vi "_Read - no objects.vi"() -> ()   [LabVIEW 2017]
uses:
  Global/GPIB Numbers.vi
  <vilib>/regexp/Match Regular Expression.xnode
panel:
  out "error out":errorcluster
  in  "Input Setting":dbl
  in  "Sensitivity":i8
  out "X, Y, and R array":dbl[](array[numeric])
  in  "error in (no error)":errorcluster
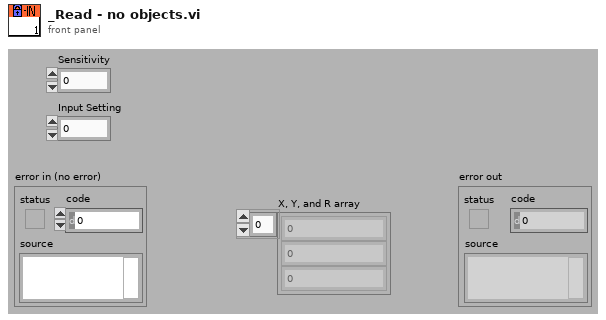
[diagram p1: front panel]
types:
  T1 = typedef "GPIB Type Def.ctl" = cluster{"Name":string, "bus":dbl, "GPIB":dbl, "GPIB as string":string, "byte":i32, "VISA Resource Name":refnum<visa-resource-name>}
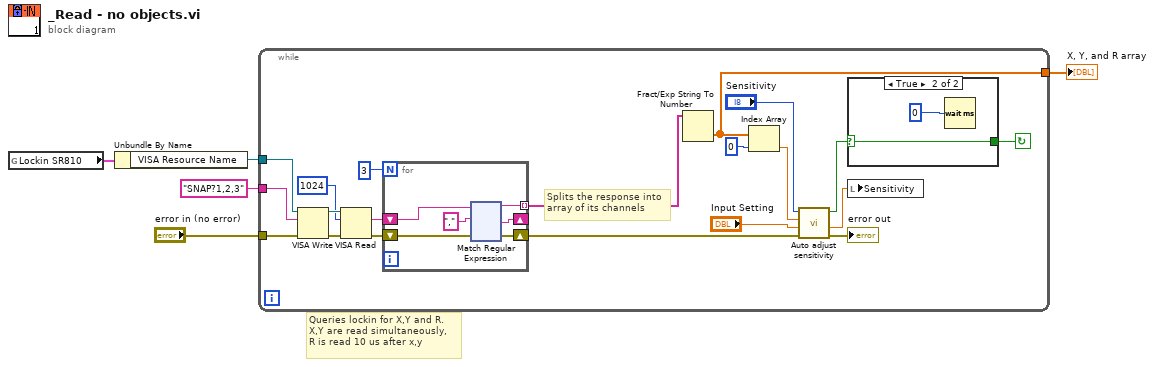
[diagram p0: block diagram]
diagram:
  # "Queries lockin for X,Y and R.\nX,Y are read simultaneously, \nR is read 10 us after x,y"
  n1 = global read "GPIB Numbers.vi" "Lockin SR810"() -> (w4:T1)
  n2 = Unbundle By Name(w4) -> ("VISA Resource Name"=w3:refnum<visa-resource-name>)
  n3 = while {
    tunnel: "SNAP?1,2,3" ("write buffer") -> [w25]
    tunnel: w3 -> [w17]
    tunnel: "error in (no error)" -> [w18]
    tunnel: [w15] -> w1
    stop <- w8 continue-if-true
    # "Splits the response into\narray of its channels"
    n4 = VISA Write(VISA resource name=w17, write buffer=w25, error in (no error)=w18) -> (VISA resource name out=w21:refnum<visa-resource-name>, error out=w20:errorcluster)  [unwired: 1 out]
    n5 = VISA Read(VISA resource name=w21, byte count=1024, error in (no error)=w20) -> (read buffer=w24:string, error out=w23:errorcluster)  [unwired: 2 out]
    n6 = for {
      N: 3 -> [_]
      tunnel: [w33] -> w16 mode=indexing
      shift-right: [w32] -> _
      shift-left: w24 -> [w31]
      shift-right: [w29] -> w7
      shift-left: w23 -> [w30]
      n7 = xnode "Match Regular Expression"("input string"=w31, "regular expression"=",", "error in"=w30) -> ("before match"=w33:string, "after match"=w32:string, "error out"=w29:errorcluster)  [unwired: 3 in, 2 out]
    }
    n8 = Fract/Exp String To Number(string=w16) -> (number=w15:dbl[])  [unwired: 3 in, 1 out]
    n9 = Index Array(array=w15, index=0) -> (element=w13:dbl)
    n10 = call "Auto adjust sensitivity.vi"("error in (no error)"=w7, "Input Setting"="Input Setting", "X value"=w13, "Sensitivity"="Sensitivity") -> ("error out"=→"error out":errorcluster, "New Sensitivity"=w12:dbl, "Repeat Measurement"=w9:bool)  [unwired: 5 in]
    n11 = case shown="True" w9 {
      selector: w9 -> [w26 w27]
      tunnel: [w26 w27] -> w8
      frame False {
      }
      frame True {
        n12 = Wait (ms)(milliseconds to wait=0) -> ()  [unwired: 1 out]
      }
    }
    n13 = local write "Sensitivity"(w12) -> ()
  }
  "X, Y, and R array" <- w1
